vi "lcr tune.vi"() -> ()   [LabVIEW 2018]
uses:
  <vilib>/DAQmx/write.llb/DAQmx Write (Analog DBL 1Chan 1Samp).vi
  2a3dda8a-b8aa-4613-8376-8d8c81e86704.vi
  <vilib>/DAQmx/read.llb/DAQmx Read (Analog DBL 1Chan 1Samp).vi
  <vilib>/Analysis/baseanly.llb/Mean (DBL).vi
  <vilib>/DAQmx/create/channels.llb/DAQmx Create Channel (AO-Voltage-Basic).vi
  <vilib>/DAQmx/miscellaneous.llb/DAQmx Fill In Error Info.vi
  <vilib>/DAQmx/create/channels.llb/DAQmx Create Channel (AI-Voltage-Basic).vi
  <vilib>/ptbypt/NI_PtbyPt.lvlib
  <vilib>/Analysis/NI_AALBase.lvlib
panel:
  out "threshold":dbl
  out "LCR Input Low":dbl=3.316831683168317
  out "LCR Input High":dbl=3.7623762376237626
  out "XY Graph 2":cluster{dbl[], dbl[]}(graph)={[0.0, 0.04950495049504951, 0.09900990099009901, 0.14851485148514854, 0.19801980198019803, 0.24752475247524752, 0.29702970297029707, 0.34653465346534656, 0.39603960396039606, 0.44554455445544555, 0.49504950495049505, 0.5445544554455446, 0.5940594059405941, 0.6435643564356436, 0.6930693069306931, 0.7425742574257426, 0.7920792079207921, 0.8415841584158417, 0.8910891089108911, 0.9405940594059407, 0.9900990099009901, 1.0396039603960396, 1.0891089108910892, 1.1386138613861387, 1.1881188118811883, 1.2376237623762376, 1.2871287128712872, 1.3366336633663367, 1.3861386138613863, 1.4356435643564358, 1.4851485148514851, 1.5346534653465347, 1.5841584158415842, 1.6336633663366338, 1.6831683168316833, 1.7326732673267327, 1.7821782178217822, 1.8316831683168318, 1.8811881188118813, 1.9306930693069309, 1.9801980198019802, 2.0297029702970297, 2.0792079207920793, 2.128712871287129, 2.1782178217821784, 2.227722772277228, 2.2772277227722775, 2.326732673267327, 2.3762376237623766, 2.4257425742574257, 2.4752475247524752, 2.5247524752475248, 2.5742574257425743, 2.623762376237624, 2.6732673267326734, 2.722772277227723, 2.7722772277227725, 2.821782178217822, 2.8712871287128716, 2.9207920792079207, 2.9702970297029703, 3.01980198019802, 3.0693069306930694, 3.118811881188119, 3.1683168316831685, 3.217821782178218, 3.2673267326732676, 3.316831683168317, 3.3663366336633667, 3.415841584158416, 3.4653465346534653, 3.514851485148515, 3.5643564356435644, 3.613861386138614, 3.6633663366336635, 3.712871287128713, 3.7623762376237626, 3.811881188118812, 3.8613861386138617, 3.9108910891089113, 3.9603960396039604, 4.00990099009901, 4.0594059405940595, 4.108910891089109, 4.158415841584159, 4.207920792079208, 4.257425742574258, 4.306930693069307, 4.356435643564357, 4.405940594059406, 4.455445544554456, 4.504950495049505, 4.554455445544555, 4.6039603960396045, 4.653465346534654, 4.702970297029704, 4.752475247524753, 4.801980198019802, 4.851485148514851, 4.900990099009901, 4.9504950495049505, 5.0], [3.6269698987299557, 3.6364573449364106, 3.6329899671345474, 3.6282543529705342, 3.629159309363951, 3.6287473758170243, 3.6300350736155056, 3.629924792216151, 3.6336451685832807, 3.63122870790565, 3.6250464609928272, 3.6300902143756275, 3.637209853485964, 3.6333467600149016, 3.630025342964688, 3.6329121214483715, 3.6278326887176044, 3.6270445008971244, 3.6230613953263267, 3.630712980049897, 3.6313000664504536, 3.6289971308177837, 3.6302329315360238, 3.6329153650017383, 3.6294609615211413, 3.63600000136827, 3.627411024462163, 3.6284100444363565, 3.6275861772915365, 3.6304729557761015, 3.629473935783759, 3.63204933151817, 3.6254162280427176, 3.627398050221512, 3.6295193457817647, 3.6331878249951624, 3.6319941907248854, 3.6278034965744808, 3.6220396703232898, 3.6262952359408596, 3.6273688580229018, 3.6348777256768994, 3.6264476837299795, 3.633719770708133, 3.6360843342001994, 3.6295290764943395, 3.6302459057692227, 3.6275504979969018, 3.6291366044222984, 3.632672097159256, 3.6235057645788302, 3.6296361143819986, 3.6328342757014656, 3.6316990257371065, 3.62449829739106, 3.629097681502316, 3.624031223133673, 3.6252702673373305, 3.6278229579737187, 3.6336192199758655, 3.6273623709287937, 3.621828838189813, 3.631844986473933, 3.625150255217819, 3.625172960190463, 3.6291917451084803, 3.6294479872235597, 3.619243711878944, 3.6345630992469626, 3.6295615122275064, 3.6293896029595634, 3.6309984143274994, 3.6328083271841956, 3.6245664123692127, 3.6280954180164486, 3.627754843002688, 3.6386662170654303, 3.62156935249656, 3.6349231357495135, 3.637310404233228, 3.6250724094892646, 3.6337684242639474, 3.638114809914663, 3.625224857360931, 3.6308427229410554, 3.637796939897928, 3.6351177500173657, 3.6332105299869375, 3.632360714266952, 3.635607529201048, 3.6308200179121477, 3.634835559237383, 3.6350820706466345, 3.6253027030898712, 3.633823564980328, 3.623252765981493, 3.6300156121881697, 3.6215855703379147, 3.6359124249670454, 3.630398353613972, 3.6265287730372937, 3.6269212451486847]}
  out "estimated polarization":dbl
  in  "background intensity":dbl
  in  "polarimeter angle":dbl
  in  "pressure factor":dbl
  in  "laser tune voltage":dbl=3.79 min=0.0 max=4.0 step=0.01
  out "Current Voltage":dbl=5.0
  # "This VI sweeps the LCR driving voltage.   LCR slow axis should be aligned to roughly 45 degrees from the \ntransmission axis of the linear plarizer.  The max and min of graph represent citical values such as 1/4 wave,\n3/4 wave, etc.  The corresponding Voltages are then used fine tune the alignemnt and to make polarization\nmeasurements."
  # "X"
  # "Y"
  # "(ignore for background measurements)"
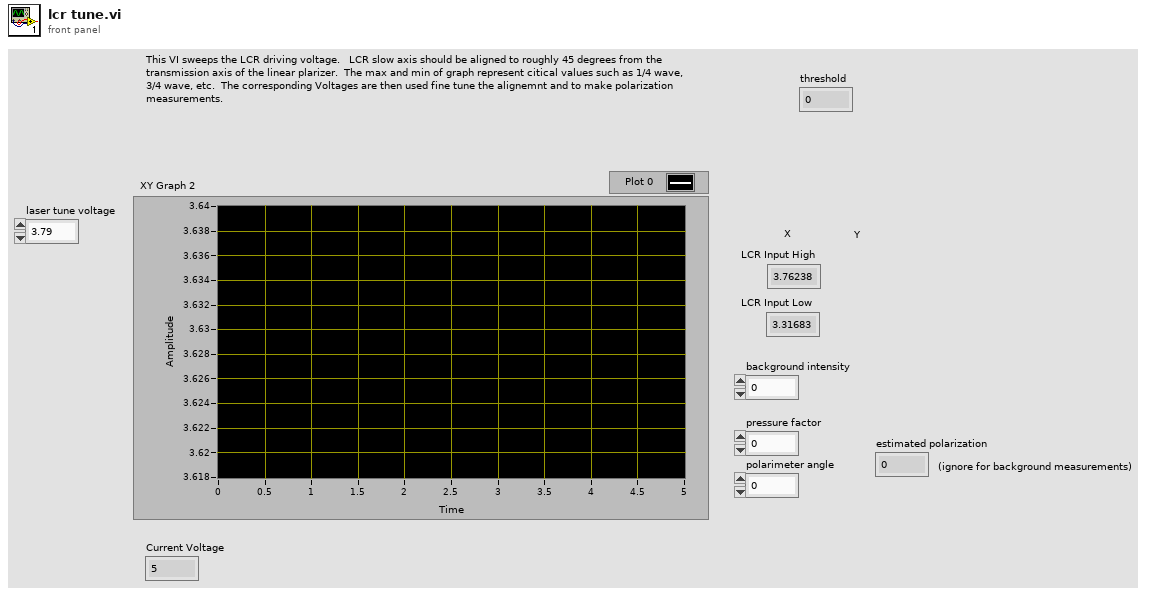
[diagram p1: front panel]
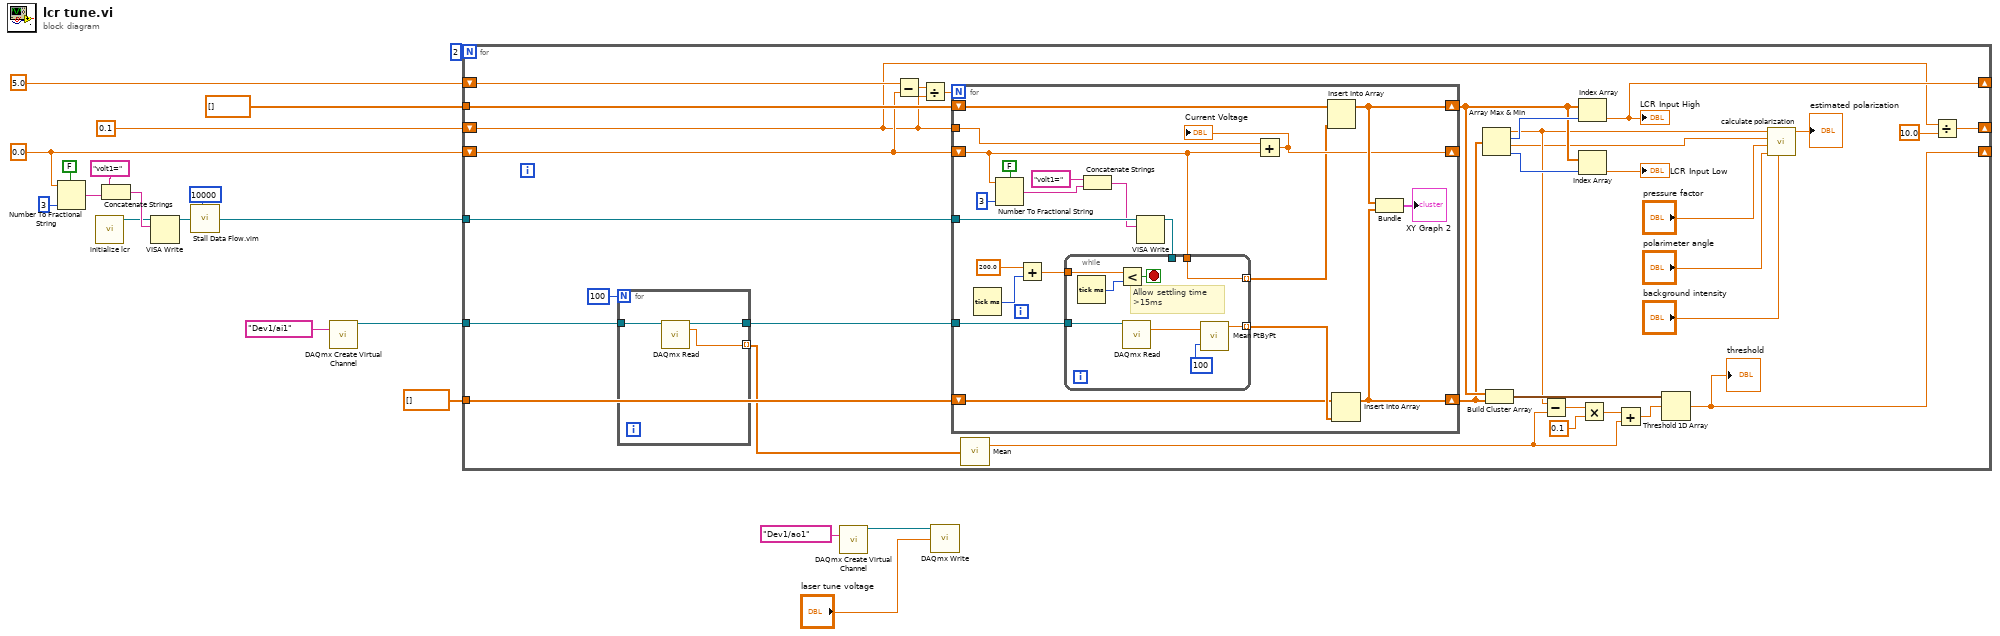
[diagram p0: block diagram]
diagram:
  w5 = 0.0 ("Start Voltage")
  n1 = Number To Fractional String(use system decimal point (T)=FALSE, number=w5, precision (6)=i16 3) -> (F-format string=w18:string)  [unwired: 1 in]
  n2 = call "initialize lcr.vi"() -> ("VISA resource name out"=w6:refnum<visa-resource-name>)  [unwired: 11 in]
  n3 = Concatenate Strings("volt1=" ("string"), w18) -> (w16:string)
  n4 = VISA Write(VISA resource name=w6, write buffer=w16) -> (VISA resource name out=w8:refnum<visa-resource-name>)  [unwired: 1 in, 2 out]
  n5 = call "Stall Data Flow.vim"("value in"=w8, "milliseconds to wait"=u32 10000) -> ("value out"=w7:refnum<visa-resource-name>)  [unwired: 1 out]
  n6 = call-poly <vilib>:"DAQmx Create Virtual Channel.vi"("physical channels"=tag "Dev1/ai1") -> ("task out"=w1:refnum<k21>)  [unwired: 13 in, 1 out]
  n7 = for {
    N: 2 -> [_]
    tunnel: dbl[] [] -> [w53]
    tunnel: dbl[] [] -> [w52]
    tunnel: w7 -> [w24]
    shift-right: [w29] -> _
    shift-left: 0.1 ("step size") -> [w28]
    shift-right: [w30] -> _
    shift-left: w5 -> [w32]
    shift-right: [w31] -> _
    shift-left: 5.0 ("End Voltage") -> [w34]
    tunnel: w1 -> [w21]
    n8 = for {
      N: 100 -> [_]
      tunnel: [w56] -> w23
      tunnel: [w55] -> w22 mode=indexing
      tunnel: w21 -> [w54]
      n9 = call-poly <vilib>:"DAQmx Read.vi"("task/channels in"=w54) -> ("task out"=w56:refnum<k21>, "data"=w55:dbl)  [unwired: 12 in, 1 out]
    }
    n10 = Subtract(x=w34, y=w32) -> (x-y=w33:dbl)
    n11 = Divide(x=w33, y=w28) -> (x/y=w35:dbl)
    n12 = for {
      N: w35 -> [_]
      tunnel: w24 -> [w73]
      shift-right: [w59] -> _
      shift-left: w32 -> [w58]
      tunnel: w28 -> [w63]
      tunnel: w23 -> [w71]
      shift-right: [w61] -> w42
      shift-left: w53 -> [w64]
      shift-right: [w62] -> w43
      shift-left: w52 -> [w65]
      n13 = Tick Count (ms)() -> (millisecond timer value=w70:u32)
      n14 = Number To Fractional String(use system decimal point (T)=FALSE, number=w58, precision (6)=i16 3) -> (F-format string=w75:string)  [unwired: 1 in]
      n15 = Add(x=200.0 ("Step length (ms)"), y=w70) -> (x+y=w68:dbl)
      n16 = Concatenate Strings("volt1=" ("string"), w75) -> (w72:string)
      n17 = VISA Write(VISA resource name=w73, write buffer=w72) -> (VISA resource name out=w67:refnum<visa-resource-name>)  [unwired: 1 in, 2 out]
      n18 = while {
        tunnel: w71 -> [w85]
        tunnel: w68 -> [w84]
        tunnel: w67 -> [_]
        tunnel: [w79] -> w66 mode=indexing
        tunnel: w58 -> [w78]
        tunnel: [w78] -> w57 mode=indexing
        stop <- w82 stop-if-true
        # "Allow settling time\n>15ms"
        n19 = Tick Count (ms)() -> (millisecond timer value=w83:u32)
        n20 = Less?(x=w84, y=w83) -> (x < y?=w82:bool)
        n21 = call-poly <vilib>:"DAQmx Read.vi"("task/channels in"=w85) -> ("data"=w81:dbl)  [unwired: 12 in, 2 out]
        n22 = call <vilib>:"Mean PtByPt.vi"("x"=w81, "sample length"=100) -> ("mean"=w79:dbl)  [unwired: 2 in, 1 out]
      }
      n23 = Add(x=w63, y=w58) -> (x+y=w59:dbl)
      "Current Voltage" <- w59
      n24 = Insert Into Array(array=w65, new element=w57) -> (w62:dbl[])  [unwired: 1 in]
      n25 = Insert Into Array(array=w64, new element=w66) -> (w61:dbl[])  [unwired: 1 in]
      n26 = Bundle(w62, w61) -> (→"XY Graph 2":cluster{dbl[], dbl[]})  [unwired: 1 in]
    }
    n27 = call-poly <vilib>:"Mean.vi"("X"=w22) -> ("mean"=w26:dbl)  [unwired: 1 out]
    n28 = Array Max & Min(array=w42) -> (max value=w41:dbl, max index (indices)=w46:i32, min value=w36:dbl, min index (indices)=w45:i32)
    n29 = Build Cluster Array(w43, w42) -> (w48:cluster{dbl, "mean":dbl}[])
    n30 = Subtract(x=w41, y=w26) -> (x-y=w49:dbl)
    n31 = Index Array(array=w43, index=w46) -> (element=w31:dbl)
    "LCR Input High" <- w31
    n32 = Index Array(array=w43, index=w45) -> (element=→"LCR Input Low":dbl)
    n33 = Multiply(x=w49, y=0.1) -> (x*y=w50:dbl)
    n34 = Add(x=w50, y=w26) -> (x+y=w51:dbl)
    n35 = Threshold 1D Array(2:w51, 3:w48) -> (0:w30:dbl)  [unwired: 1 in]
    "threshold" <- w30
    n36 = call "calculate polarization.vi"("background intensity"="background intensity", "polarimeter angle"="polarimeter angle", "pressure factor"="pressure factor", "min"=w36, "max"=w41) -> ("estimated polarization"=→"estimated polarization":dbl)  [unwired: 6 in]
    n37 = Divide(x=w28, y=10.0) -> (x/y=w29:dbl)
  }
  n38 = call-poly <vilib>:"DAQmx Create Virtual Channel.vi"("physical channels"=tag "Dev1/ao1") -> ("task out"=w9:refnum<k21>)  [unwired: 13 in, 1 out]
  n39 = call-poly <vilib>:"DAQmx Write.vi"("task/channels in"=w9, "data"="laser tune voltage") -> ()  [unwired: 11 in, 3 out]
